vi "SD Read Boolean Rarely.vi"(11 "Name":string="Numeric") -> (1 "Boolean":bool)   [LabVIEW 2013]
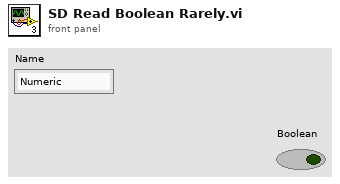
[diagram p1: front panel]
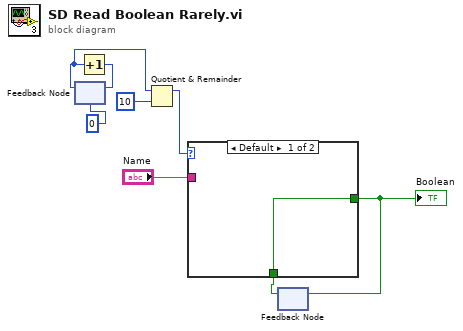
[diagram p0: block diagram]
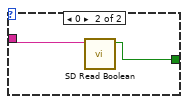
[diagram p2: hidden frame]
diagram:
  n1 = feedback #1(0) -> (w1:i32)
  n2 = Increment(x=w1) -> (x+1=w6:i32)
  n3 = feedback-in #1(w6) -> ()
  n4 = Quotient & Remainder(x=w1, y=10) -> (x-y*floor(x/y)=w4:i32)  [unwired: 1 out]
  n5 = feedback #2() -> (w2:bool)  [unwired: 1 in]
  n6 = case shown="Default" w4 {
    tunnel: "Name" -> [_ w11]
    tunnel: [w9 w10] -> w3
    tunnel: w2 -> [w9 _]
    frame Default {
    }
    frame 0 {
      n7 = call <vilib>:"SD Read Boolean.vi"("Name"=w11) -> ("Boolean"=w10:bool)  [unwired: 8 in, 2 out]
    }
  }
  "Boolean" <- w3
  n8 = feedback-in #2(w3) -> ()
